vi "Get Msgs.vi"(11 "Msgs in":refnum<class "Get Msgs.lvclass">) -> (2 "Msgs":T1)   [LabVIEW 2020, in "jettl.lvlib" / "Get Msgs.lvclass"]
uses:
  Get Msgs.lvclass
  Actor/Msgs.ctl
  Msg/Msg.lvclass
  Actor/Actor.lvlib
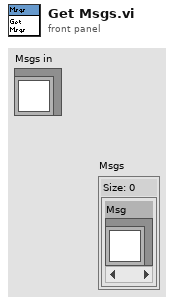
[diagram p1: front panel]
types:
  T1 = typedef "jettl.lvlib/Actor.lvlib/Msgs.ctl" = set{refnum<class "Msg.lvclass">}
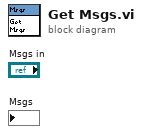
[diagram p0: block diagram]
diagram:
